vi "Instrument Get On Station.vi"(8 "error in (no error)":errorcluster, 10 "Station Record":T3, 11 "Connection Refnum":T2) -> (0 "error out":errorcluster, 2 "Instruments on Station":T1[](array[typedef]), 3 "Connection Refnum":T2, 4 "Data Present?":bool)   [LabVIEW 2011]
uses:
  Station Record.ctl
  SI.LIB/ODBC/SQL Controls/Connection Refnum.ctl
  Instrument Record.ctl
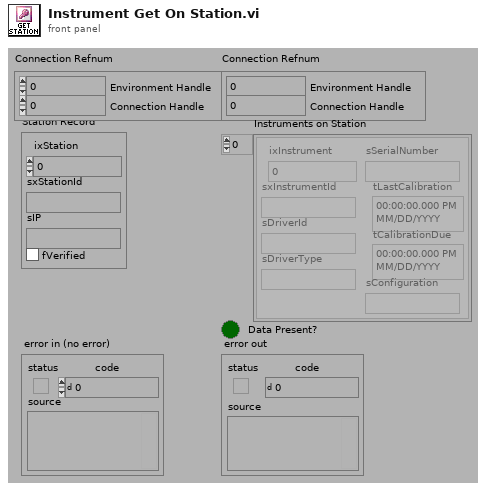
[diagram p1: front panel]
types:
  T1 = typedef "Instrument Record.ctl" = cluster{"ixInstrument":i32, "sxInstrumentId":string, "sDriverId":string, "sDriverType":string, "sSerialNumber":string, "tLastCalibration":timestamp, "tCalibrationDue":timestamp, "sConfiguration":string}
  T2 = typedef "Connection Refnum.ctl" = cluster{"Environment Handle":i32, "Connection Handle":i32}
  T3 = typedef "Station Record.ctl" = cluster{"ixStation":i32, "sxStationId":string, "sIP":string, "fVerified":bool}
  T4 = typedef "Association Record.ctl" = cluster{"ixAssociation":i32, "iStation":i32, "iInstrument":i32}
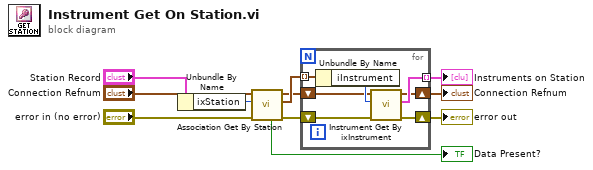
[diagram p0: block diagram]
diagram:
  n1 = Unbundle By Name("Station Record") -> ("ixStation"=w6:i32)
  n2 = call "Association Get By Station.vi"("error in (no error)"="error in (no error)", "iStation (0)"=w6, "Connection Refnum"="Connection Refnum") -> ("error out"=w7:errorcluster, "Associations"=w10:T4[], "Connection Refnum"=w8:T2, "Data Present?"=→"Data Present?":bool)  [unwired: 5 out]
  n3 = for {
    tunnel: w10 -> [w18] mode=indexing
    tunnel: [w17] -> w9 mode=indexing
    shift-right: [w14] -> w4
    shift-left: w8 -> [w15]
    shift-right: [w12] -> w3
    shift-left: w7 -> [w13]
    n4 = Unbundle By Name(w18) -> ("iInstrument"=w16:i32)
    n5 = call "Instrument Get By ixInstrument.vi"("error in (no error)"=w13, "ixInstrument"=w16, "Connection Refnum"=w15) -> ("error out"=w12:errorcluster, "Instrument Record"=w17:T1, "Connection Refnum"=w14:T2)  [unwired: 6 out]
  }
  "error out" <- w3
  "Connection Refnum" <- w4
  "Instruments on Station" <- w9
